vi "PV Diaphragm Pumps Set value settings.vi"(8 "error in (no error)":errorcluster, 10 "Adress of unit":u16=1 min=1 max=999 step=1, 11 "VISA session":refnum<visa-resource-name>) -> (0 "error out":errorcluster, 2 "response (data)":string, 3 "dup VISA session":refnum<visa-resource-name>)   [LabVIEW 2021, in "Pfeiffer Vacuum.lvlib"]
doc: "There are 4 parameters available, only one of which can be enabled at a time. \n\nSetpoint in speed setting mode [707]\nSetpoint speed in standby operation [717]\nSetting for purge gas activ [721]\nRS-485 interface address [797]\n\nNote: The controls right of this one will set the appropriate values for the selected parameter. Any settings for an parameter that is not selected will be ignored. If a value is out of range, it will be changed to either the upper or the lower limit of the range."
uses:
  <instrlib>/Pfeiffer Vacuum/Pfeiffer Vacuum.lvlib
  <instrlib>/Pfeiffer Vacuum/Public/DiaphragmPumps/PV Diapdragm Pumps Set value settings - Cluster.ctl
panel:
  in  "MVP Diaphragm Pumps Set value settings - Cluster":T1={"Parameter"=enum."Setpoint in speed setting mode [707]", "Parameter\nread only<->describe"=FALSE, "Setpoint in speed setting mode [707]"=50.0, "Setpoint speed in standby operation [717]"=66.0, "Setting for purge gas activ [721]"=3600, "Unit adress"=1} caption="Operating adjustment - Cluster" {"Setting for purge gas activ [721]" min=6 max=3600 step=1; "Unit adress" min=1 max=255 step=1; "Setpoint speed in standby operation [717]" min=20.0 max=100.0 step=0.1 format="%.2f"; "Setpoint in speed setting mode [707]" min=20.0 max=100.0 step=0.1 format="%.2f"}
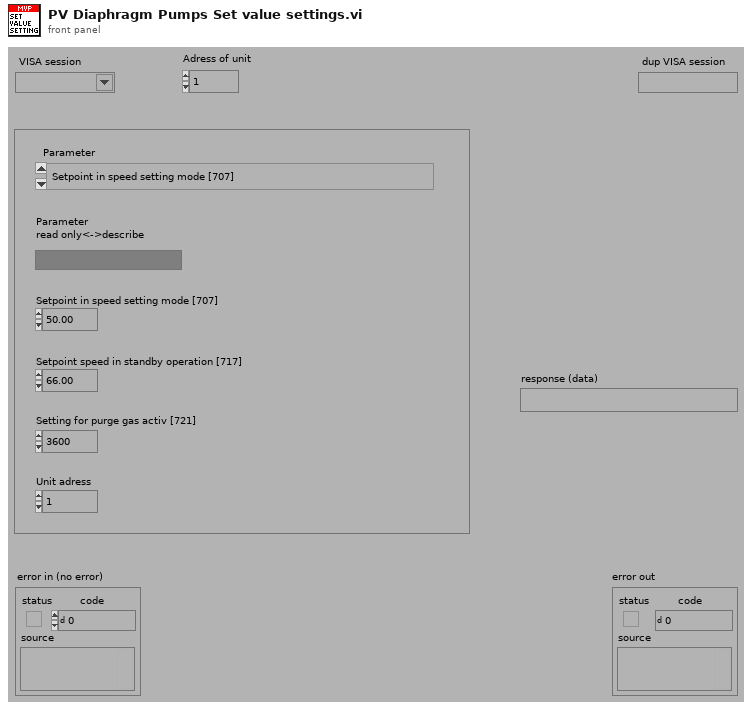
[diagram p1: front panel]
types:
  T1 = typedef "Pfeiffer Vacuum.lvlib/PV Diapdragm Pumps Set value settings - Cluster.ctl" = cluster{"Parameter":enum16{"Setpoint in speed setting mode [707]", "Setpoint speed in standby operation [717]", "Setting for purge gas activ [721]", "RS-485 interface address [797]"}, "Parameter\nread only<->describe":bool, "Setpoint in speed setting mode [707]":dbl, "Setpoint speed in standby operation [717]":dbl, "Setting for purge gas activ [721]":u16, "Unit adress":i16}
  T2 = enum16{"Setpoint in speed setting mode [707]", "Setpoint speed in standby operation [717]", "Setting for purge gas activ [721]", "RS-485 interface address [797]"}
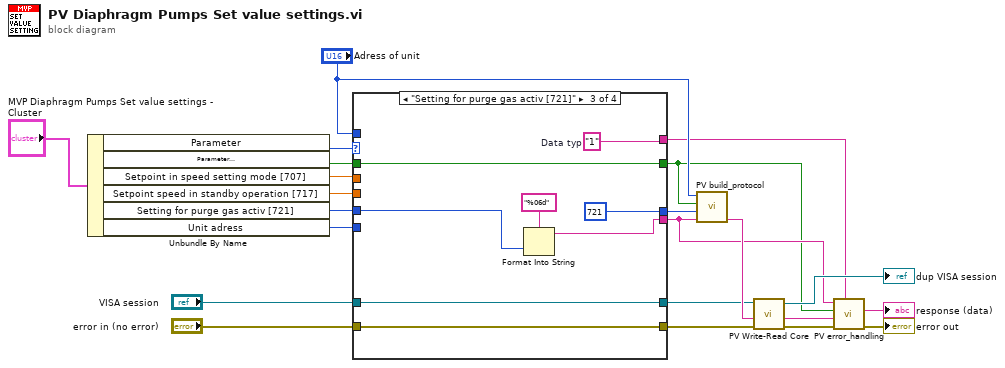
[diagram p0: block diagram]
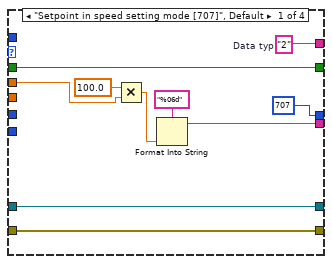
[diagram p2: hidden frame]
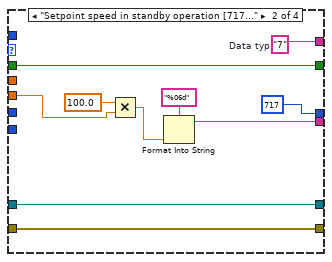
[diagram p3: hidden frame]
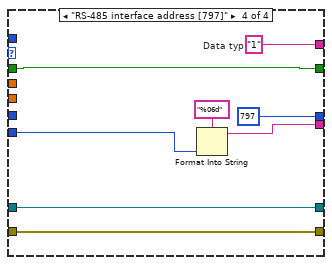
[diagram p4: hidden frame]
diagram:
  n1 = Unbundle By Name("MVP Diaphragm Pumps Set value settings - Cluster") -> ("Parameter"=w21:T2, "Parameter\nread only<->describe"=w20:bool, "Setpoint in speed setting mode [707]"=w4:dbl, "Setpoint speed in standby operation [717]"=w3:dbl, "Setting for purge gas activ [721]"=w2:u16, "Unit adress"=w1:i16)
  n2 = case shown="\"Setting for purge gas activ [721]\"" w21 {
    tunnel: [u16 707 ("Parameter-number") u16 717 ("Parameter-number") u16 721 ("Parameter-number") u16 797 ("Parameter-number")] -> w22
    tunnel: [w24 w34 w45 w53] -> w10
    tunnel: [w27 w36 w43 w52] -> w8
    tunnel: w20 -> [w27 w36 w43 w52]
    tunnel: w4 -> [w23 _ _ _]
    tunnel: w3 -> [_ w33 _ _]
    tunnel: [w26 w37 w47 w51] -> w9
    tunnel: "VISA session" -> [w32 w42 w50 w58]
    tunnel: [w32 w42 w50 w58] -> w15
    tunnel: "Adress of unit" -> [_ _ _ _]
    tunnel: "error in (no error)" -> [w31 w41 w49 w57]
    tunnel: [w31 w41 w49 w57] -> w14
    tunnel: w2 -> [_ _ w44 _]
    tunnel: w1 -> [_ _ _ w55]
    frame "Setpoint in speed setting mode [707]", Default {
      w26 = "2"  # Data typ
      n3 = Multiply(x=100.0, y=w23) -> (x*y=w29:dbl)
      n4 = Format Into String(format string="%06d" ("Format-String"), w29) -> (resulting string=w24:string)  [unwired: 2 in, 1 out]
    }
    frame "Setpoint speed in standby operation [717]" {
      w37 = "7"  # Data typ
      n5 = Multiply(x=100.0, y=w33) -> (x*y=w39:dbl)
      n6 = Format Into String(format string="%06d" ("Format-String"), w39) -> (resulting string=w34:string)  [unwired: 2 in, 1 out]
    }
    frame "Setting for purge gas activ [721]" {
      w47 = "1"  # Data typ
      n7 = Format Into String(format string="%06d" ("Format-String"), w44) -> (resulting string=w45:string)  [unwired: 2 in, 1 out]
    }
    frame "RS-485 interface address [797]" {
      w51 = "1"  # Data typ
      n8 = Format Into String(format string="%06d" ("Format-String"), w55) -> (resulting string=w53:string)  [unwired: 2 in, 1 out]
    }
  }
  n9 = call <instrlib>:"PV build_protocol.vi"("Data"=w10, "Parameter-number"=w22, "parameter\nread<->describe"=w8, "Adress"="Adress of unit") -> ("output"=w16:string)  [unwired: 3 in]
  n10 = call <instrlib>:"PV Write-Read Core.vi"("error in"=w14, "Write data in"=w16, "VISA session"=w15) -> ("error out"=w12:errorcluster, "response (data) out"=w13:string, "dup VISA session"=→"dup VISA session":refnum<visa-resource-name>)  [unwired: 2 in]
  n11 = call <instrlib>:"PV error_handling.vi"("Data Typ in"=w9, "error in"=w12, "response (data) in"=w13, "Parameter\nread only<->describe"=w8, "data in"=w10) -> ("error out"=→"error out":errorcluster, "Data out"=→"response (data)":string)  [unwired: 4 in, 1 out]
